vi "CRYO_VavleControlProto_2.vi"() -> ()   [LabVIEW 2017]
uses:
  <vilib>/DAQmx/miscellaneous.llb/DAQmx Fill In Error Info.vi
  <vilib>/DAQmx/create/channels.llb/DAQmx Create Channel (DO-Digital Output).vi
panel:
  in  "Ctrl 2":bool
  in  "DAQ DOUT ch1 2":tag="Dev1/port1/line1"
  out "V2 Status":T1(ring)=enum."OPEN"
  in  "Ctrl 1":bool
  out "V1 Status":T1(ring)=enum."CLOSED"
  out "DOUT task out":refnum<k21>="20200907_142127_DO"
  in  "DAQ DOUT ch1":tag="Dev1/port1/line0"
  in  "Stop Button":bool
  out "Error Out":errorcluster
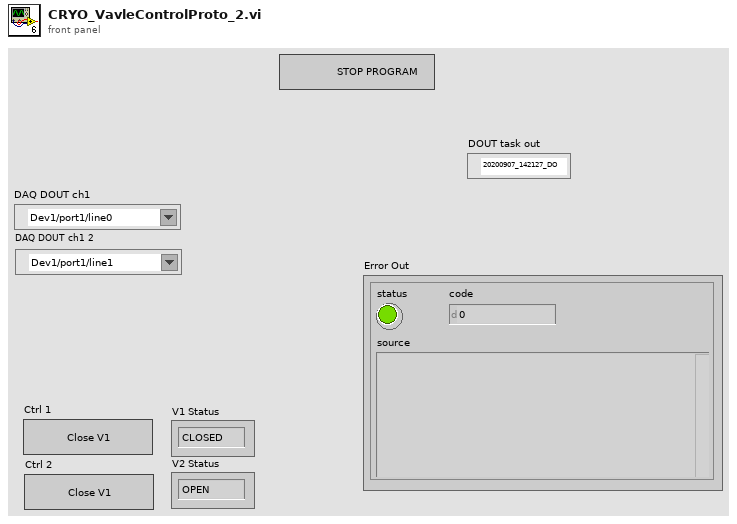
[diagram p1: front panel]
types:
  T1 = enum16{"Initialzied", "OPEN", "CLOSED", "Undefined", ""}
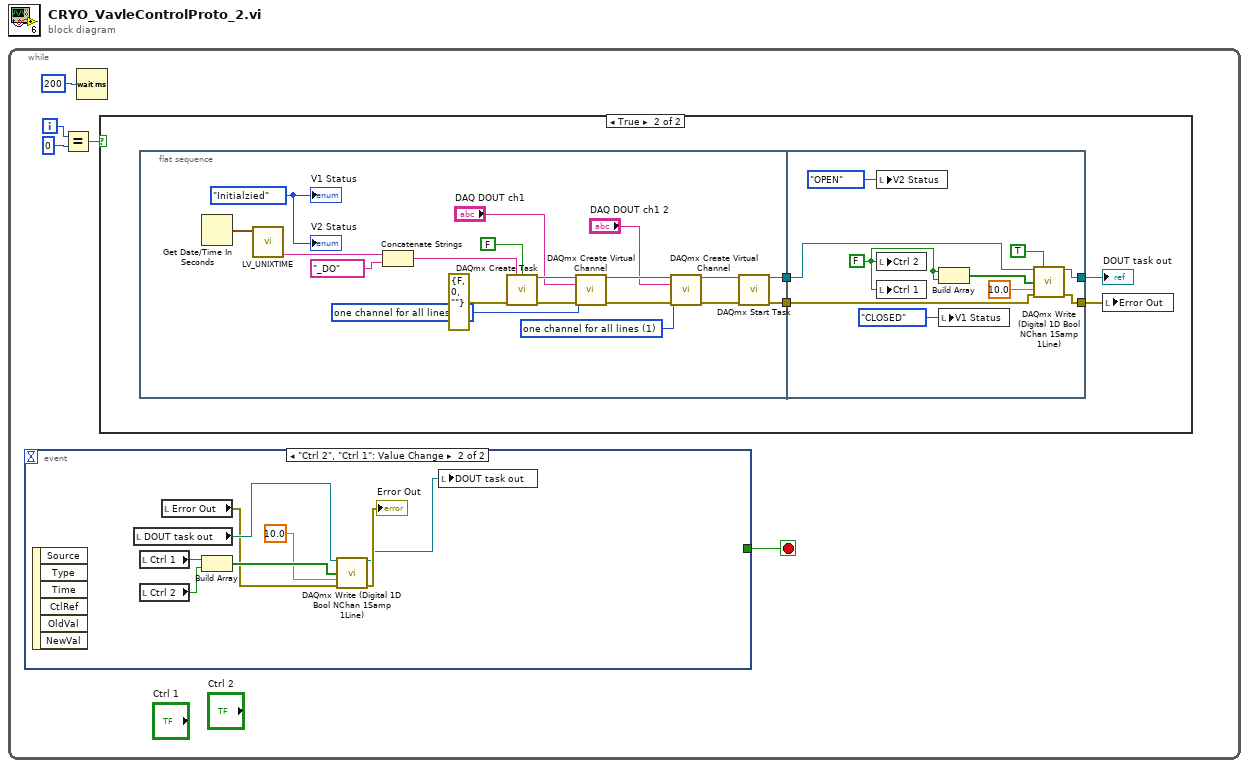
[diagram p0: block diagram]
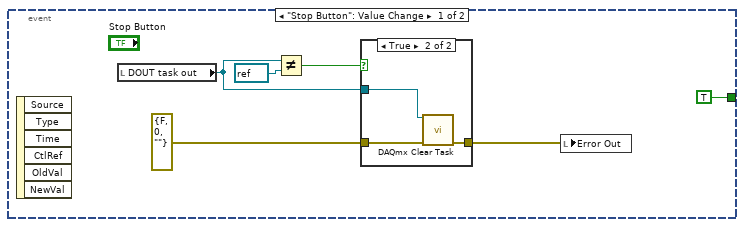
[diagram p3: hidden frame]
diagram:
  n1 = while {
    i -> [w3]
    stop <- w4 stop-if-true
    n2 = event shown="[1] \"Ctrl 2\", \"Ctrl 1\": Value Change" {
      selector: _ -> [_ _]
      dyn-events: _ -> [_ _]
      timeout: _ -> [_ _]
      tunnel: [TRUE ("Stop Button") _] -> w4
      event "Stop Button": Value Change {
        n3 = event-data() -> ()  [unwired: 1 in, 6 out]
        n4 = local read "DOUT task out"() -> (w43:refnum<k21>)
        n5 = Not Equal?(x=w43, y=refnum<k21> refnum ("AO task out")) -> (x != y?=w42:bool)
        n6 = case shown="True" w42 {
          tunnel: w43 -> [_ w48]
          tunnel: [w45 w47] -> w39
          tunnel: errorcluster {"status"=FALSE, "code"=0, "source"=""} ("error in") -> [w45 w46]
          frame False {
          }
          frame True {
            n7 = call <vilib>:"DAQmx Clear Task.vi"("task in"=w48, "error in"=w46) -> ("error out"=w47:errorcluster)  [unwired: 13 in]
          }
        }
        n8 = local write "Error Out"(w39) -> ()
      }
      event "Ctrl 2", "Ctrl 1": Value Change {
        n9 = event-data() -> ()  [unwired: 1 in, 6 out]
        n10 = local read "DOUT task out"() -> (w54:refnum<k21>)
        n11 = local read "Ctrl 1"() -> (w56:bool)
        n12 = local read "Ctrl 2"() -> (w55:bool)
        n13 = local read "Error Out"() -> (w51:errorcluster)
        n14 = Build Array(w56, w55) -> (w53:bool[])
        n15 = call <vilib>:"DAQmx Write (Digital 1D Bool NChan 1Samp 1Line).vi"("task/channels in"=w54, "data"=w53, "timeout"=10.0, "error in"=w51) -> ("task out"=w49:refnum<k21>, "error out"=→"Error Out":errorcluster)  [unwired: 9 in, 1 out]
        n16 = local write "DOUT task out"(w49) -> ()
      }
    }
    n17 = Equal?(x=w3, y=0) -> (x = y?=w1:bool)
    n18 = Wait (ms)(milliseconds to wait=u32 200) -> ()  [unwired: 1 out]
    n19 = case shown="True" w1 {
      frame False {
      }
      frame True {
        n20 = flat-sequence {
          tunnel: [w24] -> w8
          tunnel: [w12] -> w7
          tunnel: [w29] -> w9
          tunnel: w8 -> [w30]
          tunnel: w7 -> [w33]
          tunnel: [w35] -> w6
          frame #0 {
            w10 = 1 items=["one channel for each line", "one channel for all lines"] ("line grouping")
            w11 = 1 items=["one channel for each line", "one channel for all lines"] ("line grouping")
            w13 = T1."Initialzied" ("V2 Status")
            n21 = Get Date/Time In Seconds() -> (seconds since 1Jan1904=w21:timestamp)
            n22 = call "LV_UNIXTIME.vi"("current time"=w21) -> ("date/time string"=w20:string)  [unwired: 9 in, 1 out]
            n23 = Concatenate Strings(w20, "_DO" ("new task name")) -> (w27:string)
            n24 = call <vilib>:"DAQmx Create Task.vi"("new task name"=w27, "auto cleanup"=FALSE, "error in"=errorcluster {"status"=FALSE, "code"=0, "source"=""}) -> ("task out"=w26:refnum<k21>, "error out"=w25:errorcluster)  [unwired: 11 in]
            n25 = call-poly <vilib>:"DAQmx Create Virtual Channel.vi"("task in"=w26, "lines"="DAQ DOUT ch1", "line grouping"=w10, "error in"=w25) -> ("task out"=w18:refnum<k21>, "error out"=w17:errorcluster)  [unwired: 10 in]
            n26 = call-poly <vilib>:"DAQmx Create Virtual Channel.vi"("task in"=w18, "lines"="DAQ DOUT ch1 2", "line grouping"=w11, "error in"=w17) -> ("task out"=w14:refnum<k21>, "error out"=w16:errorcluster)  [unwired: 10 in]
            n27 = call <vilib>:"DAQmx Start Task.vi"("task/channels in"=w14, "error in"=w16) -> ("task out"=w12:refnum<k21>, "error out"=w24:errorcluster)  [unwired: 12 in]
            "V1 Status" <- w13
            "V2 Status" <- w13
          }
          frame #1 {
            w36 = FALSE ("Ctrl 2")
            n28 = local write "V2 Status"(T1."OPEN" ("V2 Status")) -> ()
            n29 = local write "Ctrl 2"(w36) -> ()
            n30 = local write "Ctrl 1"(w36) -> ()
            n31 = Build Array(w36, w36) -> (w32:bool[])
            n32 = local write "V1 Status"(T1."CLOSED" ("V1 Status")) -> ()
            n33 = call <vilib>:"DAQmx Write (Digital 1D Bool NChan 1Samp 1Line).vi"("task/channels in"=w33, "auto start"=TRUE, "data"=w32, "timeout"=10.0, "error in"=w30) -> ("task out"=w35:refnum<k21>, "error out"=w29:errorcluster)  [unwired: 8 in, 1 out]
          }
        }
        n34 = local write "Error Out"(w9) -> ()
        "DOUT task out" <- w6
      }
    }
  }
